vi "Get adas_GetStatusResponse.vi"(8 "error in (no error)":errorcluster, 11 "gRPCid":T2) -> (0 "error out":errorcluster, 2 "package_templatemessage":T1, 3 "gRPCid out":T2)   [LabVIEW 2023, in "BLSClimateChamberTemplateService_server.lvlib"]
uses:
  BLSClimateChamberTemplateService_server.lvlib
  <vilib>/gRPC/LabVIEW gRPC Library/Shared/grpcId.ctl
  adas_GetStatusResponse.ctl
  a51dd2a7-b5c1-4c09-9df4-8cd9d3bd0c19.vi
  <vilib>/gRPC/LabVIEW gRPC Library/Shared/TranslateGrpcError.vi
  <vilib>/gRPC/LabVIEW gRPC Library/Server API/Server/Get Server DLL Path.vi
  <vilib>/Utility/error.llb/Error Cluster From Error Code.vi
  <vilib>/gRPC/LabVIEW gRPC Library/grpc-lvsupport-release.lvlib
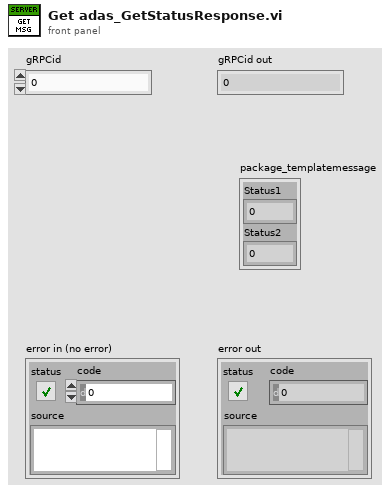
[diagram p1: front panel]
types:
  T1 = typedef "BLSClimateChamberTemplateService_server.lvlib/adas_GetStatusResponse.ctl" = cluster{"Status1":u32, "Status2":u32}
  T2 = typedef "grpc-lvsupport-release.lvlib/grpcId.ctl" = u64
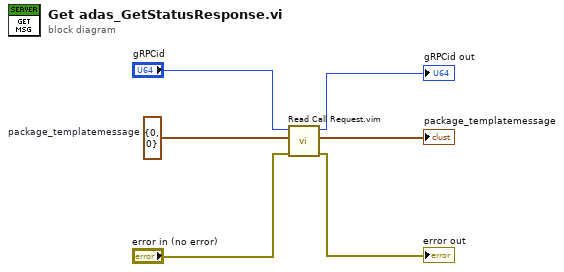
[diagram p0: block diagram]
diagram:
  w2 = T1 {"Status1"=0, "Status2"=0}  # package_templatemessage
  n1 = call "Read Call Request.vim"("error in"="error in (no error)", "Request Type"=w2, "gRPCid in"="gRPCid") -> ("error out"=→"error out":errorcluster, "Request Data"=→"package_templatemessage":T1, "gRPCid out"=→"gRPCid out":T2)  [unwired: 6 in]
